vi "Init.vi"() -> (0 "error out":errorcluster, 2 "output cluster":T15, 3 "OpenSuccesfull":bool, 5 "Motor & Solonoid Cluster":cluster{T18[], T26[]}, 6 "PixySPIDevRef":T16={"DevStatus"={"status"=FALSE, "code"=0, "source"=""}, "Handle"=0, "Controller"=enum."Controller 1", "SPI Bus"=enum."Invalid"})   [LabVIEW 2014]
uses:
  <vilib>/Rock Robotics/WPI/MotorControl/WPI_MotorControlDeviceRef.ctl
  <vilib>/Rock Robotics/WPI/MotorControl/WPI_MotorControlType.ctl
  <vilib>/Rock Robotics/SystemInterfaces/Typedef/FPGA_TypedefDigitalModule.ctl
  <vilib>/Rock Robotics/SystemInterfaces/DIO/FPGA_DIOPWMChannel.ctl
  <vilib>/Rock Robotics/WPI/PWM/WPI_PWMDeadband.ctl
  <vilib>/Rock Robotics/WPI/CAN/Jaguar/SubVIs/WPI_CANJaguar_ControlMode.ctl
  <vilib>/Rock Robotics/WPI/CAN/TalonSRX/WPI_CANTalonSRX_APIControlMode.ctl
  <vilib>/Rock Robotics/WPI/PWM/WPI_PWMTransform_ConPane.ctl
  <vilib>/Rock Robotics/WPI/Solenoid/WPI_SolenoidDevRef.ctl
  <vilib>/Rock Robotics/WPI/Solenoid/WPI_SolenoidChannel.ctl
  <vilib>/Rock Robotics/WPI/SPI/WPI_SPIDevRef.ctl
  <vilib>/Rock Robotics/SystemInterfaces/spilib/spi_bus.ctl
  <vilib>/Rock Robotics/WPI/Joystick/WPI_JoystickDevRef.ctl
  <vilib>/Rock Robotics/WPI/Joystick/WPI_JoystickDeviceEnum.ctl
  <vilib>/Rock Robotics/WPI/Potentiometer/WPI_PotentiometerDevRef.ctl
  <vilib>/Rock Robotics/SystemInterfaces/Typedef/FPGA_TypedefAnalogModule.ctl
  <vilib>/Rock Robotics/SystemInterfaces/AI/FPGA_AIChannel.ctl
  <vilib>/Rock Robotics/WPI/Encoder/WPI_EncoderDevRef.ctl
  <vilib>/Rock Robotics/SystemInterfaces/Encoder/FPGA_EncoderIdx.ctl
  <vilib>/Rock Robotics/SystemInterfaces/Counter/FPGA_CounterCtrSystemIndex.ctl
  <vilib>/Rock Robotics/WPI/Encoder/WPI_EncoderType.ctl
  <vilib>/Rock Robotics/WPI/Switch/WPI_SwitchDevRef.ctl
  <vilib>/Rock Robotics/SystemInterfaces/DIO/FPGA_DIOChannel.ctl
  <vilib>/Rock Robotics/WPI/Gyro/WPI_GyroDevRef.ctl
  <vilib>/Rock Robotics/WPI/Compressor/WPI_CompressorDevRef.ctl
  <vilib>/Rock Robotics/SystemInterfaces/AI/FPGA_AIGyroChannel.ctl
  <vilib>/Rock Robotics/WPI/MotorControl/WPI_MotorControlOpen VictorSP.vi
  <vilib>/Rock Robotics/WPI/Counter/WPI_CounterDigitalInputToDigitalSource.vi
  <vilib>/Rock Robotics/WPI/Solenoid/WPI_SolenoidOpenSingle.vi
  <vilib>/Rock Robotics/WPI/Switch/WPI_SwitchOpenLimit.vi
  Peripherals/Nav6Library/Nav6.lvlib
  <vilib>/Rock Robotics/WPI/SPI/WPI_SPIMode.ctl
panel:
  out "Calibrated Center Voltage Out":dbl
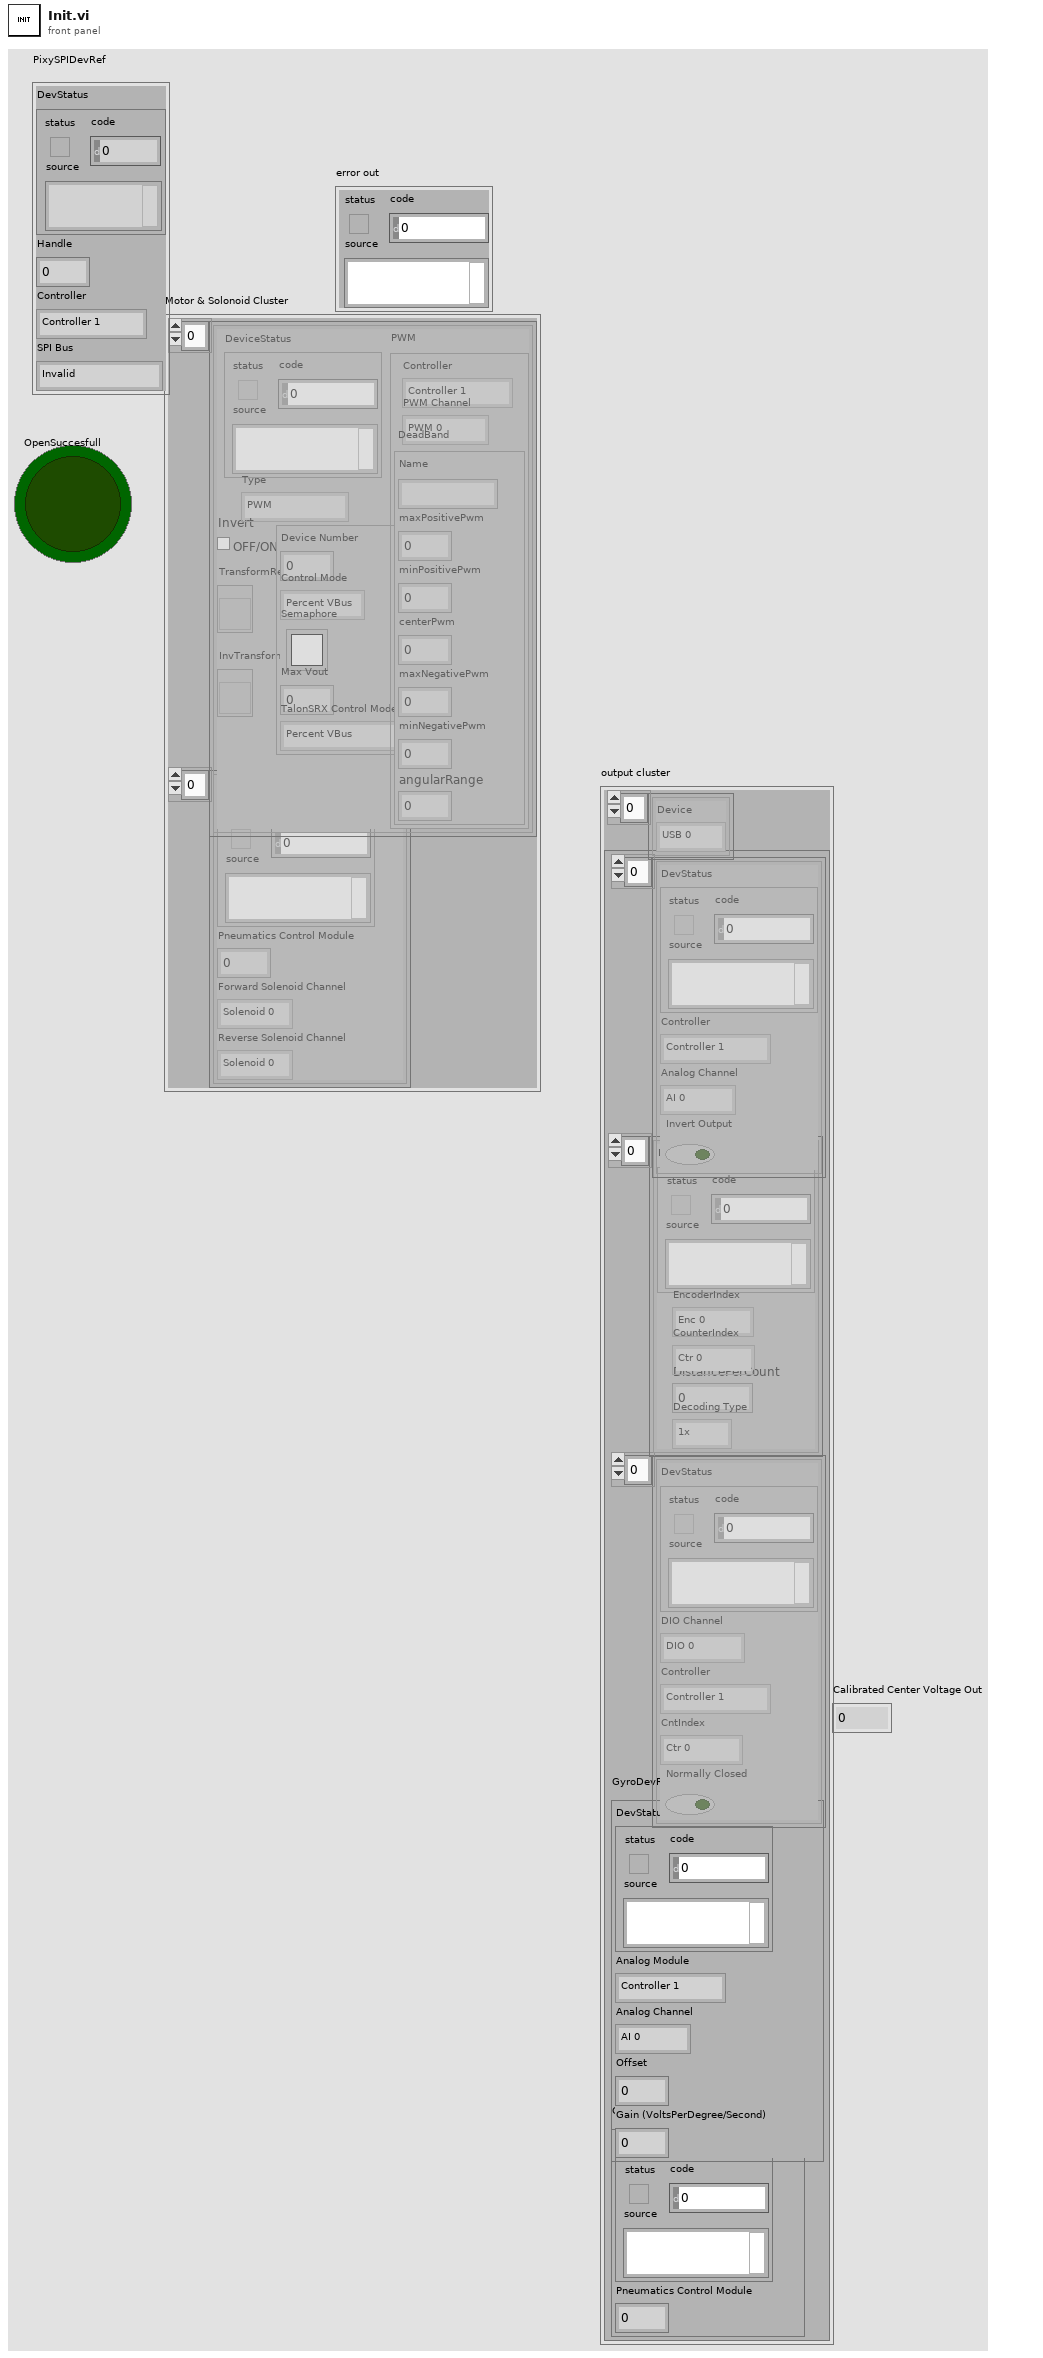
[diagram p1: front panel]
types:
  T1 = typedef "WPI_JoystickDevRef.ctl" = cluster{"Device":T2}
  T2 = typedef "WPI_JoystickDeviceEnum.ctl" = enum16{"USB 0", "USB 1", "USB 2", "USB 3", "USB 4", "USB 5"}
  T3 = typedef "WPI_PotentiometerDevRef.ctl" = cluster{"DevStatus":errorcluster, "Controller":T4, "Analog Channel":T5, "Invert Output":bool}
  T4 = typedef "FPGA_TypedefAnalogModule.ctl" = enum16{"Controller 1"}
  T5 = typedef "FPGA_AIChannel.ctl" = enum8{"AI 0", "AI 1", "AI 2", "AI 3", "AI MXP 0", "AI MXP 1", "AI MXP 2", "AI MXP 3", "Invalid"}
  T6 = typedef "WPI_EncoderDevRef.ctl" = cluster{"DevStatus":errorcluster, "EncoderIndex":T7, "CounterIndex":T8, "DistancePerCount":dbl, "Decoding Type":T9}
  T7 = typedef "FPGA_EncoderIdx.ctl" = enum8{"Enc 0", "Enc 1", "Enc 2", "Enc 3", "Enc 4", "Enc 5", "Enc 6", "Enc 7", "Invalid"}
  T8 = typedef "FPGA_CounterCtrSystemIndex.ctl" = enum8{"Ctr 0", "Ctr 1", "Ctr 2", "Ctr 3", "Ctr 4", "Ctr 5", "Ctr 6", "Ctr 7", "Invalid"}
  T9 = typedef "WPI_EncoderType.ctl" = enum16{"1x", "2x", "4x"}
  T10 = typedef "WPI_SwitchDevRef.ctl" = cluster{"DevStatus":errorcluster, "DIO Channel":T11, "Controller":T12, "CntIndex":T8, "Normally Closed":bool}
  T11 = typedef "FPGA_DIOChannel.ctl" = enum8{"DIO 0", "DIO 1", "DIO 2", "DIO 3", "DIO 4", "DIO 5", "DIO 6", "DIO 7", "DIO 8", "DIO 9", "DIO MXP 0", "DIO MXP 1", "DIO MXP 2", "DIO MXP 3", "DIO MXP 4", "DIO MXP 5", "DIO MXP 6", "DIO MXP 7", "DIO MXP 8", "DIO MXP 9", "DIO MXP 10", "DIO MXP 11", "DIO MXP 12", "DIO MXP 13", "DIO MXP 14", "DIO MXP 15", "Invalid"}
  T12 = typedef "FPGA_TypedefDigitalModule.ctl" = enum16{"Controller 1"}
  T13 = typedef "WPI_GyroDevRef.ctl" = cluster{"DevStatus":errorcluster, "Analog Module":T4, "Analog Channel":T5, "Offset":dbl, "Gain (VoltsPerDegree/Second)":dbl}
  T14 = typedef "WPI_CompressorDevRef.ctl" = cluster{"DevStatus":errorcluster, "Pneumatics Control Module":u8}
  T15 = cluster{T1[], cluster{T3[], T6[], T10[], "GyroDevRef":T13, "CompressorDevRef":T14}}
  T16 = typedef "WPI_SPIDevRef.ctl" = cluster{"DevStatus":errorcluster, "Handle":i32, "Controller":T12, "SPI Bus":T17}
  T17 = typedef "spi_bus.ctl" = enum16{"SPI On-Board, CS0", "SPI On-Board, CS1", "SPI On-Board, CS2", "SPI On-Board, CS3", "SPI MXP", "Invalid"}
  T18 = typedef "WPI_MotorControlDeviceRef.ctl" = cluster{"DeviceStatus":errorcluster, "Type":T19, "PWM":cluster{"Controller":T12, "PWM Channel":T20, "DeadBand":T21}, "CAN":cluster{"Device Number":u8, "Control Mode":T22, "Semaphore":T23, "Max Vout":dbl, "TalonSRX Control Mode":T24}, "Invert":bool, "TransformRef":T25, "InvTransformRef":T25}
  T19 = typedef "WPI_MotorControlType.ctl" = enum16{"PWM", "CAN", "CANTalonSRX"}
  T20 = typedef "FPGA_DIOPWMChannel.ctl" = enum8{"PWM 0", "PWM 1", "PWM 2", "PWM 3", "PWM 4", "PWM 5", "PWM 6", "PWM 7", "PWM 8", "PWM 9", "PWM MXP 0", "PWM MXP 1", "PWM MXP 2", "PWM MXP 3", "PWM MXP 4", "PWM MXP 5", "PWM MXP 6", "PWM MXP 7", "PWM MXP 8", "PWM MXP 9", "Invalid"}
  T21 = typedef "WPI_PWMDeadband.ctl" = cluster{"Name":string, "maxPositivePwm":i32, "minPositivePwm":i32, "centerPwm":i32, "maxNegativePwm":i32, "minNegativePwm":i32, "angularRange":u16}
  T22 = typedef "WPI_CANJaguar_ControlMode.ctl" = enum8{"Percent VBus", "Current", "Speed", "Position", "Voltage"}
  T23 = typedef "Semaphore RefNum" = refnum<k1>
  T24 = typedef "WPI_CANTalonSRX_APIControlMode.ctl" = enum8{"Percent VBus", "Speed", "Position", "Slave", "Unchanged / Invalid"}
  T25 = typedef "WPI_PWMTransform_ConPane.ctl" = refnum<vi>
  T26 = typedef "WPI_SolenoidDevRef.ctl" = cluster{"DevStatus":errorcluster, "Pneumatics Control Module":u8, "Forward Solenoid Channel":T27, "Reverse Solenoid Channel":T27}
  T27 = typedef "WPI_SolenoidChannel.ctl" = enum8{"Solenoid 0", "Solenoid 1", "Solenoid 2", "Solenoid 3", "Solenoid 4", "Solenoid 5", "Solenoid 6", "Solenoid 7", "Invalid"}
  T28 = typedef "FPGA_AIGyroChannel.ctl" = enum8{"AI 0", "AI 1", "Invalid"}
  T29 = typedef "WPI_SerialPortRef.ctl" = cluster{"DevStatus":errorcluster, "Serial Port Name":refnum<visa-resource-name>}
  T30 = typedef "Nav6.lvlib/Nav6DevRef.ctl" = cluster{"SerialPortRef":T29, "UpdateRate":u8, "Error":errorcluster, "Nav6Mode":T31}
  T31 = typedef "Nav6.lvlib/Nav6Mode.ctl" = enum16{"YPR", "Gyro", "Quaternion"}
  T32 = typedef "WPI_SPIMode.ctl" = enum16{"Mode 0 (Clk Idle Low,Sample on Leading)", "Mode 1 (Clk Idle Low,Sample on Trailing)", "Mode 2 (Clk Idle High,Sample on Leading)", "Mode 3 (Clk Idle High,Sample on Trailing)"}
  T33 = typedef "WPI_DigitalInputDevRef.ctl" = cluster{"DevStatus":errorcluster, "DIO Channel":T11, "Controller":T12}
  T34 = typedef "FPGA_CounterEncoderSourceConvertionLVSourceType.ctl" = cluster{"DevStatus":errorcluster, "AnalogTriggerMode?":bool, "DigitalMode":cluster{"Controller":T12, "DIO Channel":T35}, "AnalogTriggerMode":cluster{"AnalogTriggerIndex":T36, "OutputType":T37}}
  T35 = typedef "FPGA_DIODigitalSourceChannel.ctl" = enum8{"DIO 0", "DIO 1", "DIO 2", "DIO 3", "DIO 4", "DIO 5", "DIO 6", "DIO 7", "DIO 8", "DIO 9", "DIO MXP 0", "DIO MXP 1", "DIO MXP 2", "DIO MXP 3", "DIO MXP 4", "DIO MXP 5", "DIO MXP 6", "DIO MXP 7", "DIO MXP 8", "DIO MXP 9", "DIO MXP 10", "DIO MXP 11", "DIO MXP 12", "DIO MXP 13", "DIO MXP 14", "DIO MXP 15", "Disabled"}
  T36 = typedef "FPGA_AnalogTriggerIndex.ctl" = enum8{"Trig 0", "Trig 1", "Trig 2", "Trig 3", "Trig 4", "Trig 5", "Trig 6", "Trig 7", "Invalid"}
  T37 = typedef "FPGA_AnalogTriggerOutType.ctl" = enum16{"InWindow", "TriggerState", "Rising", "Falling"}
  T38 = cluster{T3[], T6[], T10[], "GyroDevRef":T13, "CompressorDevRef":T14}
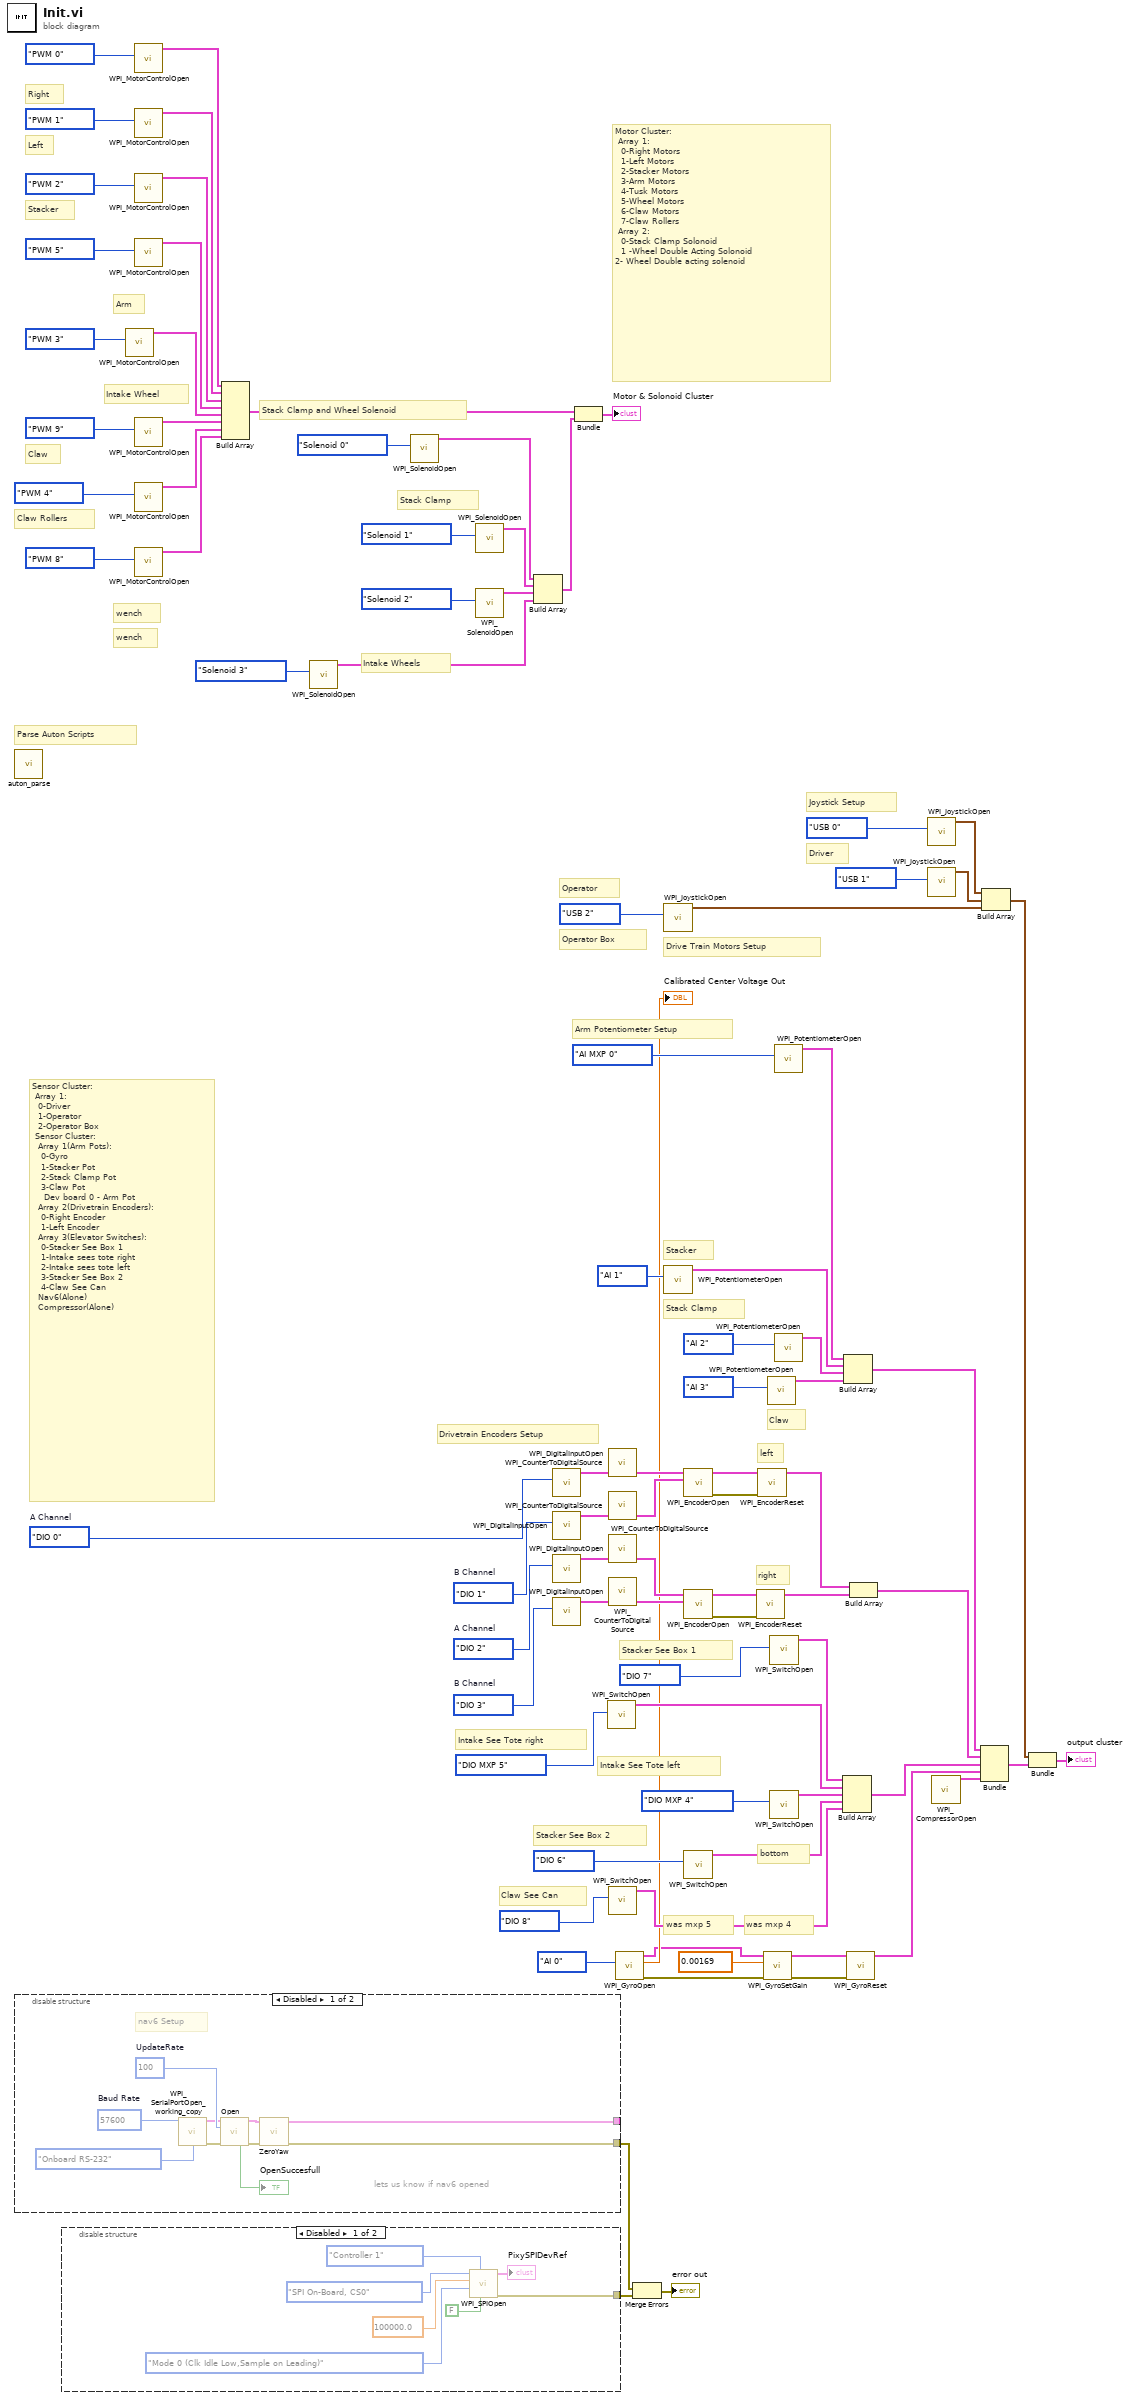
[diagram p0: block diagram]
diagram:
  w75 = FPGA_DIOChannel."DIO 3"  # B Channel
  w74 = FPGA_DIOChannel."DIO 2"  # A Channel
  w81 = FPGA_DIOChannel."DIO 1"  # B Channel
  w80 = FPGA_DIOChannel."DIO 0"  # A Channel
  # "wench"
  # "wench"
  # "was mxp 4"
  # "was mxp 5"
  # "Claw Rollers"
  # "Claw"
  # "Claw See Can"
  # "Claw"
  # "Intake Wheels"
  # "Stack Clamp"
  # "Intake See Tote left"
  # "Intake See Tote right"
  # "Stacker See Box 2"
  # "Sensor Cluster:\n Array 1:\n  0-Driver\n  1-Operator\n  2-Operator Box\n Sensor Cluster:\n  Array 1(Arm Pots):\n   0-Gyro\n   1-Stacker Pot\n   2-Stack Clamp Pot\n   3-Claw Pot\n    Dev board 0 - Arm Pot\n  Array 2(Drivetrain Encoders):\n   0-Right Encoder\n   1-Left Encoder\n  Array 3(Elevator Switches):\n   0-Stacker See Box 1\n   1-Intake sees tote right\n   2-Intake sees tote left\n   3-Stacker See Box 2\n   4-Claw See Can \n  Nav6(Alone)\n  Compressor(Alone)"
  # "Stacker"
  # "Stacker See Box 1"
  # "bottom"
  # "right"
  # "left"
  # "Stack Clamp"
  # "Intake Wheel"
  # "Operator Box"
  # "Operator"
  # "Driver"
  # "Motor Cluster:\n Array 1:\n  0-Right Motors\n  1-Left Motors\n  2-Stacker Motors\n  3-Arm Motors\n  4-Tusk Motors\n  5-Wheel Motors\n  6-Claw Motors\n  7-Claw Rollers\n Array 2:\n  0-Stack Clamp Solonoid\n  1 -Wheel Double Acting Solonoid\n2- Wheel Double acting solenoid"
  # "Left"
  # "Right"
  # "Stack Clamp and Wheel Solenoid"
  # "Arm"
  # "Stacker"
  # "Drivetrain Encoders Setup"
  # "Arm Potentiometer Setup"
  # "Drive Train Motors Setup"
  # "Joystick Setup"
  # "Parse Auton Scripts"
  n1 = call "auton_parse.vi"() -> ()  [unwired: 1 in]
  n2 = disable-structure shown="Disabled" {
    disable-tunnel: [w97 _] -> _
    disable-tunnel: [w96 _] -> w17
    frame Disabled {
      w91 = u32 57600  # Baud Rate
      w95 = u8 100  # UpdateRate
      # "lets us know if nav6 opened"
      # "nav6 Setup"
      n3 = call "WPI_SerialPortOpen_working_copy.vi"("Baud Rate"=w91, "Serial Port"=enum16{"Onboard RS-232", "MXP TTL", "USB"}."Onboard RS-232") -> ("SerialPortRef"=w90:T29, "error out"=w89:errorcluster)  [unwired: 12 in]
      n4 = call "Open.vi"("SerialPortRef"=w90, "UpdateRate (100Hz)"=w95, "error in (no error)"=w89) -> ("Nav6DevRef"=w93:T30, "Open Succesfull"=→"OpenSuccesfull":bool, "error out"=w92:errorcluster)  [unwired: 6 in, 4 out]
      n5 = call "ZeroYaw.vi"("error in (no error)"=w92, "Nav6DevRef"=w93) -> ("error out"=w96:errorcluster, "Nav6DevRef Out"=w97:T30)  [unwired: 8 in]
    }
    frame Enabled {
    }
  }
  n6 = disable-structure shown="Disabled" {
    disable-tunnel: [w99 _] -> w16
    frame Disabled {
      n7 = call <vilib>:"WPI_SPIOpen.vi"("Chip Select Active High (F)"=FALSE, "Controller"=FPGA_TypedefDigitalModule."Controller 1", "Mode (3)"=WPI_SPIMode."Mode 0 (Clk Idle Low,Sample on Leading)", "Clock Rate (Hz)"=100000.0, "SPI Bus"=spi_bus."SPI On-Board, CS0") -> ("error out"=w99:errorcluster, "SPIDevRef"=→"PixySPIDevRef":T16)  [unwired: 5 in]
    }
    frame Enabled {
    }
  }
  n8 = call-poly <vilib>:"WPI_MotorControlOpen.vi"("PWM Channel"=FPGA_DIOPWMChannel."PWM 3") -> ("MotorControlDeviceRef"=w38:T18)  [unwired: 9 in, 1 out]
  n9 = call-poly <vilib>:"WPI_MotorControlOpen.vi"("PWM Channel"=FPGA_DIOPWMChannel."PWM 0") -> ("MotorControlDeviceRef"=w60:T18)  [unwired: 9 in, 1 out]
  n10 = call-poly <vilib>:"WPI_MotorControlOpen.vi"("PWM Channel"=FPGA_DIOPWMChannel."PWM 1") -> ("MotorControlDeviceRef"=w59:T18)  [unwired: 9 in, 1 out]
  n11 = call-poly <vilib>:"WPI_MotorControlOpen.vi"("PWM Channel"=FPGA_DIOPWMChannel."PWM 2") -> ("MotorControlDeviceRef"=w58:T18)  [unwired: 9 in, 1 out]
  n12 = call-poly <vilib>:"WPI_MotorControlOpen.vi"("PWM Channel"=FPGA_DIOPWMChannel."PWM 5") -> ("MotorControlDeviceRef"=w57:T18)  [unwired: 9 in, 1 out]
  n13 = call-poly <vilib>:"WPI_MotorControlOpen.vi"("PWM Channel"=FPGA_DIOPWMChannel."PWM 9") -> ("MotorControlDeviceRef"=w20:T18)  [unwired: 9 in, 1 out]
  n14 = call-poly <vilib>:"WPI_MotorControlOpen.vi"("PWM Channel"=FPGA_DIOPWMChannel."PWM 4") -> ("MotorControlDeviceRef"=w5:T18)  [unwired: 9 in, 1 out]
  n15 = call-poly <vilib>:"WPI_MotorControlOpen.vi"("PWM Channel"=FPGA_DIOPWMChannel."PWM 8") -> ("MotorControlDeviceRef"=w2:T18)  [unwired: 9 in, 1 out]
  n16 = Build Array(w60, w59, w58, w57, w38, w20, w5, w2) -> (w53:T18[])
  n17 = call-poly <vilib>:"WPI_SolenoidOpen.vi"("Solenoid Channel"=WPI_SolenoidChannel."Solenoid 3") -> ("SolenoidDevRef"=w3:T26)  [unwired: 9 in, 1 out]
  n18 = call-poly <vilib>:"WPI_SolenoidOpen.vi"("Solenoid Channel"=WPI_SolenoidChannel."Solenoid 0") -> ("SolenoidDevRef"=w56:T26)  [unwired: 9 in, 1 out]
  n19 = call-poly <vilib>:"WPI_SolenoidOpen.vi"("Solenoid Channel"=WPI_SolenoidChannel."Solenoid 1") -> ("SolenoidDevRef"=w55:T26)  [unwired: 9 in, 1 out]
  n20 = call-poly <vilib>:"WPI_SolenoidOpen.vi"("Solenoid Channel"=WPI_SolenoidChannel."Solenoid 2") -> ("SolenoidDevRef"=w26:T26)  [unwired: 9 in, 1 out]
  n21 = Build Array(w56, w55, w26, w3) -> (w54:T26[])
  n22 = call <vilib>:"WPI_DigitalInputOpen.vi"("DIO Channel"=w80) -> ("DigitalInputDevRef"=w77:T33)  [unwired: 2 in, 8 out]
  n23 = call <vilib>:"WPI_DigitalInputOpen.vi"("DIO Channel"=w81) -> ("DigitalInputDevRef"=w78:T33)  [unwired: 2 in, 8 out]
  n24 = call <vilib>:"WPI_DigitalInputOpen.vi"("DIO Channel"=w74) -> ("DigitalInputDevRef"=w71:T33)  [unwired: 2 in, 8 out]
  n25 = call <vilib>:"WPI_DigitalInputOpen.vi"("DIO Channel"=w75) -> ("DigitalInputDevRef"=w72:T33)  [unwired: 2 in, 8 out]
  n26 = Bundle(w53, w54) -> (→"Motor & Solonoid Cluster":cluster{T18[], T26[]})  [unwired: 1 in]
  n27 = call-poly <vilib>:"WPI_SwitchOpen.vi"("DIO Channel"=FPGA_DIOChannel."DIO MXP 5") -> ("SwitchDevRef"=w33:T10)  [unwired: 9 in, 1 out]
  n28 = call-poly <vilib>:"WPI_CounterToDigitalSource.vi"("DigitalInputDevRef"=w77) -> ("Digital Source"=w76:T34)  [unwired: 6 out]
  n29 = call-poly <vilib>:"WPI_CounterToDigitalSource.vi"("DigitalInputDevRef"=w78) -> ("Digital Source"=w79:T34)  [unwired: 6 out]
  n30 = call-poly <vilib>:"WPI_CounterToDigitalSource.vi"("DigitalInputDevRef"=w71) -> ("Digital Source"=w70:T34)  [unwired: 6 out]
  n31 = call-poly <vilib>:"WPI_CounterToDigitalSource.vi"("DigitalInputDevRef"=w72) -> ("Digital Source"=w73:T34)  [unwired: 6 out]
  n32 = call-poly <vilib>:"WPI_SwitchOpen.vi"("DIO Channel"=FPGA_DIOChannel."DIO 8") -> ("SwitchDevRef"=w22:T10)  [unwired: 9 in, 1 out]
  n33 = call <vilib>:"WPI_GyroOpen.vi"("Analog Channel"=FPGA_AIGyroChannel."AI 0") -> ("error out"=w14:errorcluster, "Calibrated Center Voltage Out"=→"Calibrated Center Voltage Out":dbl, "GyroDevRef"=w9:T13)  [unwired: 8 in]
  n34 = Merge Errors(w17, w16) -> (→"error out":errorcluster)
  n35 = call <vilib>:"WPI_JoystickOpen.vi"("JoystickDevice"=WPI_JoystickDeviceEnum."USB 2") -> ("JoystickDevRef"=w50:T1)  [unwired: 10 in]
  n36 = call <vilib>:"WPI_PotentiometerOpen.vi"("Analog Channel"=FPGA_AIChannel."AI 1") -> ("PotDevRef"=w47:T3)  [unwired: 9 in, 1 out]
  n37 = call <vilib>:"WPI_EncoderOpen.vi"("BSource"=w79, "ASource"=w76) -> ("error out"=w67:errorcluster, "EncoderDevRef"=w68:T6)  [unwired: 6 in, 2 out]
  n38 = call <vilib>:"WPI_EncoderOpen.vi"("BSource"=w73, "ASource"=w70) -> ("error out"=w65:errorcluster, "EncoderDevRef"=w66:T6)  [unwired: 6 in, 2 out]
  n39 = call-poly <vilib>:"WPI_SwitchOpen.vi"("DIO Channel"=FPGA_DIOChannel."DIO 6") -> ("SwitchDevRef"=w30:T10)  [unwired: 9 in, 1 out]
  n40 = call <vilib>:"WPI_EncoderReset.vi"("error in (no error)"=w65, "EncoderDevRef"=w66) -> ("EncoderDevRef"=w45:T6)  [unwired: 8 in, 1 out]
  n41 = call <vilib>:"WPI_EncoderReset.vi"("error in (no error)"=w67, "EncoderDevRef"=w68) -> ("EncoderDevRef"=w44:T6)  [unwired: 8 in, 1 out]
  n42 = call <vilib>:"WPI_GyroSetGain.vi"("error in (no error)"=w14, "Gain (VoltsPerDegree/Second)"=0.00169, "GyroDevRef"=w9) -> ("error out"=w12:errorcluster, "GyroDevRef"=w8:T13)  [unwired: 7 in]
  n43 = call <vilib>:"WPI_PotentiometerOpen.vi"("Analog Channel"=FPGA_AIChannel."AI 3") -> ("PotDevRef"=w25:T3)  [unwired: 9 in, 1 out]
  n44 = call-poly <vilib>:"WPI_SwitchOpen.vi"("DIO Channel"=FPGA_DIOChannel."DIO 7") -> ("SwitchDevRef"=w36:T10)  [unwired: 9 in, 1 out]
  n45 = call-poly <vilib>:"WPI_SwitchOpen.vi"("DIO Channel"=FPGA_DIOChannel."DIO MXP 4") -> ("SwitchDevRef"=w32:T10)  [unwired: 9 in, 1 out]
  n46 = call <vilib>:"WPI_PotentiometerOpen.vi"("Analog Channel"=FPGA_AIChannel."AI MXP 0") -> ("PotDevRef"=w48:T3)  [unwired: 9 in, 1 out]
  n47 = call <vilib>:"WPI_PotentiometerOpen.vi"("Analog Channel"=FPGA_AIChannel."AI 2") -> ("PotDevRef"=w29:T3)  [unwired: 9 in, 1 out]
  n48 = Build Array(w36, w33, w32, w30, w22) -> (w42:T10[])
  n49 = Build Array(w48, w47, w29, w25) -> (w46:T3[])
  n50 = call <vilib>:"WPI_GyroReset.vi"("error in (no error)"=w12, "GyroDevRef"=w8) -> ("GyroDevRef"=w10:T13)  [unwired: 8 in, 1 out]
  n51 = Build Array(w44, w45) -> (w43:T6[])
  n52 = call <vilib>:"WPI_JoystickOpen.vi"("JoystickDevice"=WPI_JoystickDeviceEnum."USB 0") -> ("JoystickDevRef"=w51:T1)  [unwired: 10 in]
  n53 = call <vilib>:"WPI_JoystickOpen.vi"("JoystickDevice"=WPI_JoystickDeviceEnum."USB 1") -> ("JoystickDevRef"=w49:T1)  [unwired: 10 in]
  n54 = call <vilib>:"WPI_CompressorOpen.vi"() -> ("CompressorDevRef"=w19:T14)  [unwired: 14 in, 1 out]
  n55 = Bundle(w46, w43, w42, "GyroDevRef"=w10, "CompressorDevRef"=w19) -> (w41:T38)  [unwired: 1 in]
  n56 = Build Array(w51, w49, w50) -> (w40:T1[])
  n57 = Bundle(w40, w41) -> (→"output cluster":T15)  [unwired: 1 in]
